vi "WriteOtherInfo.vi"(4 "error in (no error)":errorcluster, 5 "# of Entries (before)":i16, 6 "Other Info":T1 {"Equinox" format="%#.2g"; "Read Noise" format="%#.2g"; "Gain" format="%#.2g"; "Exposure Time" format="%#.2g"}, 7 "Path to FITS Header File":path) -> (0 "error out":errorcluster, 2 "# of Entries (after)":i16, 3 "Path to FITS Header File":path)   [LabVIEW 2015]
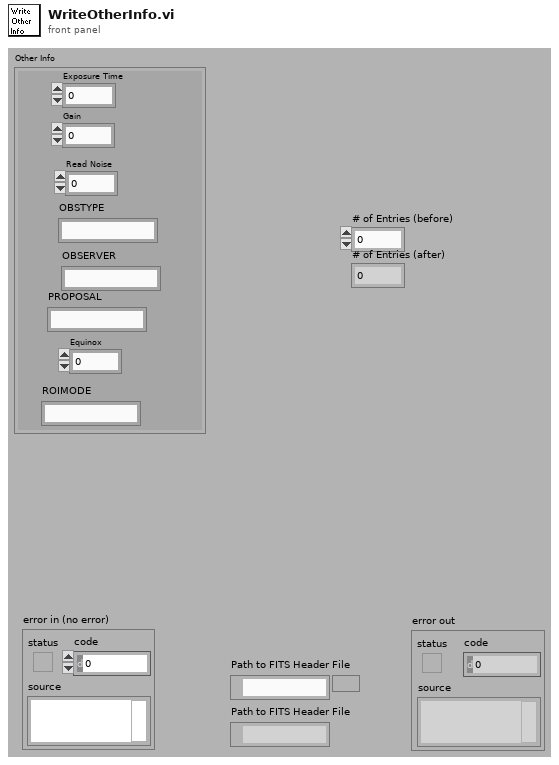
[diagram p1: front panel]
types:
  T1 = cluster{"Exposure Time":dbl, "Gain":dbl, "Read Noise":dbl, "OBSTYPE":string, "OBSERVER":string, "PROPOSAL":string, "Equinox":dbl, "ROIMODE":string}
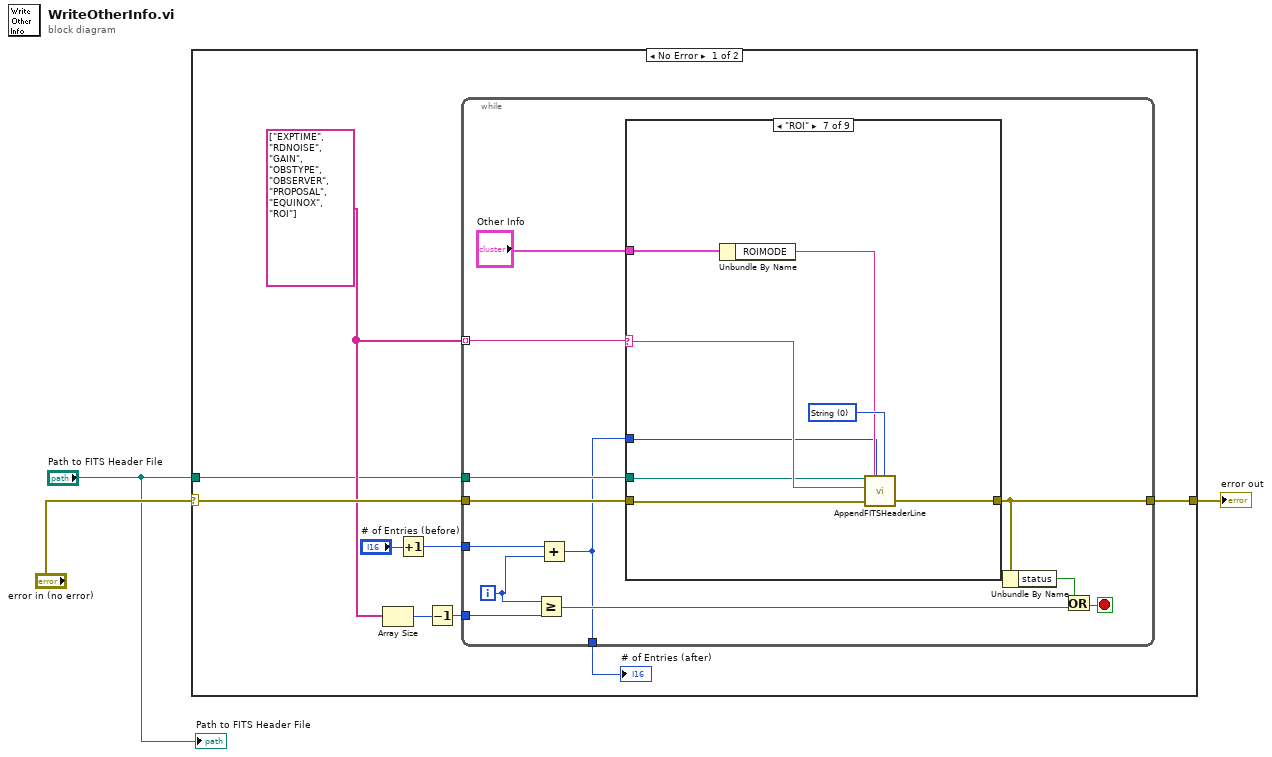
[diagram p0: block diagram]
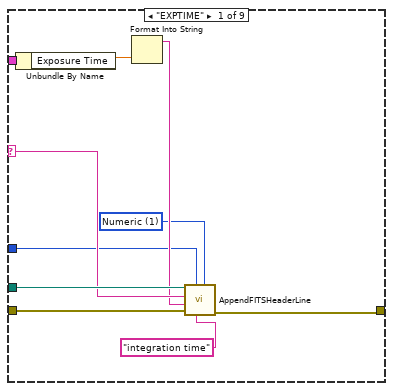
[diagram p2: hidden frame]
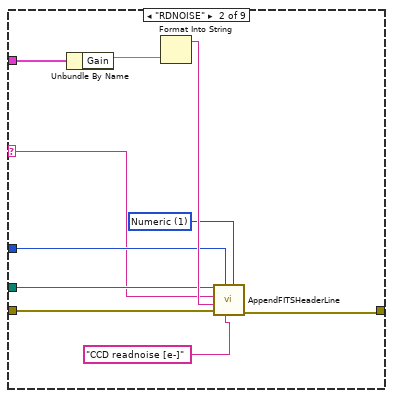
[diagram p3: hidden frame]
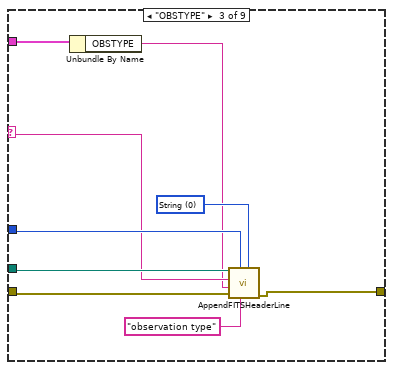
[diagram p4: hidden frame]
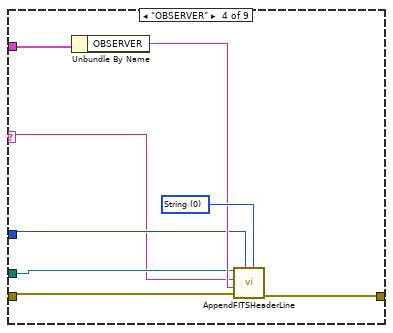
[diagram p5: hidden frame]
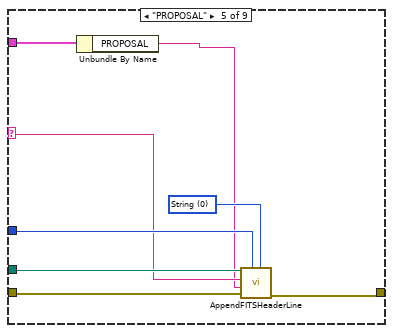
[diagram p6: hidden frame]
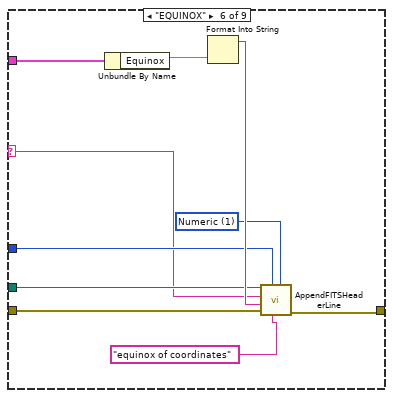
[diagram p7: hidden frame]
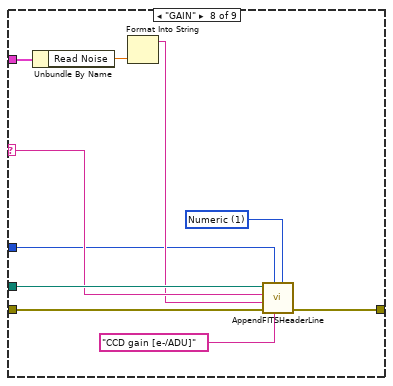
[diagram p8: hidden frame]
diagram:
  n1 = case shown="No Error" "error in (no error)" {
    selector: "error in (no error)" -> [w12 w99]
    tunnel: [w8 w99] -> w2
    tunnel: "Path to FITS Header File" -> [w7 _]
    frame No Error {
      w11 = string[] ["EXPTIME", "RDNOISE", "GAIN", "OBSTYPE", "OBSERVER", "PROPOSAL", "EQUINOX", "ROI"]
      n2 = Array Size(array=w11) -> (size(s)=w10:i32)
      n3 = Increment(x="# of Entries (before)") -> (x+1=w5:i16)
      n4 = Decrement(x=w10) -> (x-1=w9:i32)
      n5 = while {
        tunnel: w12 -> [w24]
        tunnel: w11 -> [w22] mode=indexing
        tunnel: w9 -> [w21]
        tunnel: [w20] -> w8
        tunnel: w7 -> [w16]
        tunnel: w5 -> [w14]
        tunnel: [w13] -> w4
        i -> [w15]
        stop <- w23 stop-if-true
        n6 = Greater Or Equal?(x=w15, y=w21) -> (x >= y?=w19:bool)
        n7 = Add(x=w14, y=w15) -> (x+y=w13:i32)
        n8 = case shown="\"ROI\"" w22 {
          selector: w22 -> [w31 w37 w49 w56 w65 w72 w84 w93 _]
          tunnel: w24 -> [w34 w38 w52 w59 w68 w74 w81 w96 w98]
          tunnel: [w33 w36 w46 w54 w63 w70 w80 w95 w98] -> w20
          tunnel: "Other Info" -> [w27 w41 w47 w55 w64 w71 w85 w97 _]
          tunnel: w16 -> [w32 w39 w51 w58 w67 w75 w82 w94 _]
          tunnel: w13 -> [w28 w40 w50 w57 w66 w73 w83 w89 _]
          frame "EXPTIME" {
            w29 = u16 1 items=["String", "Numeric", "Boolean"] ("Entry Type")
            n9 = Unbundle By Name(w27) -> ("Exposure Time"=w26:dbl)
            n10 = Format Into String(w26) -> (resulting string=w30:string)  [unwired: 3 in, 1 out]
            n11 = call "AppendFITSHeaderLine.vi"("Entry Type"=w29, "Comment"="integration time", "Entry #"=w28, "error in (no error)"=w34, "Element Value"=w30, "Element Name"=w31, "file path (dialog if empty)"=w32) -> ("error out"=w33:errorcluster)  [unwired: 3 in]
          }
          frame "RDNOISE" {
            w43 = u16 1 items=["String", "Numeric", "Boolean"] ("Entry Type")
            n12 = Unbundle By Name(w41) -> ("Gain"=w42:dbl)
            n13 = Format Into String(w42) -> (resulting string=w44:string)  [unwired: 3 in, 1 out]
            n14 = call "AppendFITSHeaderLine.vi"("Entry Type"=w43, "Comment"="CCD readnoise [e-]", "Entry #"=w40, "error in (no error)"=w38, "Element Value"=w44, "Element Name"=w37, "file path (dialog if empty)"=w39) -> ("error out"=w36:errorcluster)  [unwired: 3 in]
          }
          frame "OBSTYPE" {
            w53 = u16 0 items=["String", "Numeric", "Boolean"] ("Entry Type")
            n15 = Unbundle By Name(w47) -> ("OBSTYPE"=w48:string)
            n16 = call "AppendFITSHeaderLine.vi"("Entry Type"=w53, "Comment"="observation type", "Entry #"=w50, "error in (no error)"=w52, "Element Value"=w48, "Element Name"=w49, "file path (dialog if empty)"=w51) -> ("error out"=w46:errorcluster)  [unwired: 3 in]
          }
          frame "OBSERVER" {
            w61 = u16 0 items=["String", "Numeric", "Boolean"] ("Entry Type")
            n17 = Unbundle By Name(w55) -> ("OBSERVER"=w60:string)
            n18 = call "AppendFITSHeaderLine.vi"("Entry Type"=w61, "Entry #"=w57, "error in (no error)"=w59, "Element Value"=w60, "Element Name"=w56, "file path (dialog if empty)"=w58) -> ("error out"=w54:errorcluster)  [unwired: 4 in]
          }
          frame "PROPOSAL" {
            w69 = u16 0 items=["String", "Numeric", "Boolean"] ("Entry Type")
            n19 = Unbundle By Name(w64) -> ("PROPOSAL"=w62:string)
            n20 = call "AppendFITSHeaderLine.vi"("Entry Type"=w69, "Entry #"=w66, "error in (no error)"=w68, "Element Value"=w62, "Element Name"=w65, "file path (dialog if empty)"=w67) -> ("error out"=w63:errorcluster)  [unwired: 4 in]
          }
          frame "EQUINOX" {
            w78 = u16 1 items=["String", "Numeric", "Boolean"] ("Entry Type")
            n21 = Unbundle By Name(w71) -> ("Equinox"=w77:dbl)
            n22 = Format Into String(w77) -> (resulting string=w79:string)  [unwired: 3 in, 1 out]
            n23 = call "AppendFITSHeaderLine.vi"("Entry Type"=w78, "Comment"="equinox of coordinates", "Entry #"=w73, "error in (no error)"=w74, "Element Value"=w79, "Element Name"=w72, "file path (dialog if empty)"=w75) -> ("error out"=w70:errorcluster)  [unwired: 3 in]
          }
          frame "ROI" {
            w87 = u16 0 items=["String", "Numeric", "Boolean"] ("Entry Type")
            n24 = Unbundle By Name(w85) -> ("ROIMODE"=w86:string)
            n25 = call "AppendFITSHeaderLine.vi"("Entry Type"=w87, "Entry #"=w83, "error in (no error)"=w81, "Element Value"=w86, "Element Name"=w84, "file path (dialog if empty)"=w82) -> ("error out"=w80:errorcluster)  [unwired: 4 in]
          }
          frame "GAIN" {
            w90 = u16 1 items=["String", "Numeric", "Boolean"] ("Entry Type")
            n26 = Unbundle By Name(w97) -> ("Read Noise"=w92:dbl)
            n27 = Format Into String(w92) -> (resulting string=w91:string)  [unwired: 3 in, 1 out]
            n28 = call "AppendFITSHeaderLine.vi"("Entry Type"=w90, "Comment"="CCD gain [e-/ADU]", "Entry #"=w89, "error in (no error)"=w96, "Element Value"=w91, "Element Name"=w93, "file path (dialog if empty)"=w94) -> ("error out"=w95:errorcluster)  [unwired: 3 in]
          }
          frame "", Default {
          }
        }
        n29 = Unbundle By Name(w20) -> ("status"=w18:bool)
        n30 = Or(x=w18, y=w19) -> (x .or. y?=w23:bool)
      }
      "# of Entries (after)" <- w4
    }
    frame Error {
    }
  }
  "error out" <- w2
  "Path to FITS Header File" <- "Path to FITS Header File"
